vi "StringToBool.vi"(11 "StringIn":string) -> (3 "Boolean":bool)   [LabVIEW 2013, in "VariableManagerAPI.lvlib"]
doc: "Return true, if StringIn (case insensitive) is \"1\", \"T\", \"TRUE\".\nReturn false, otherwise."
uses:
  VariableManagerAPI.lvlib
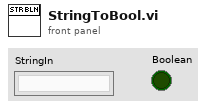
[diagram p1: front panel]
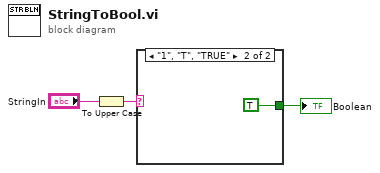
[diagram p0: block diagram]
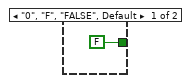
[diagram p2: hidden frame]
diagram:
  n1 = To Upper Case(1:"StringIn") -> (0:w1:string)
  n2 = case shown="\"1\", \"T\", \"TRUE\"" w1 {
    tunnel: [FALSE ("BooleanOUT") TRUE ("BooleanOUT")] -> w3
    frame "0", "F", "FALSE", Default {
    }
    frame "1", "T", "TRUE" {
    }
  }
  "Boolean" <- w3
